vi "Destroy User Events.vi"(11 "UI Template in":refnum<class "Messages Actor.lvclass">) -> (3 "UI Template out":refnum<class "Messages Actor.lvclass">)   [LabVIEW 2020, in "Messages Actor.lvlib" / "Messages Actor.lvclass"]
uses:
  Messages Actor.lvclass
  Messages Actor.lvclass/Messages Actor.ctl
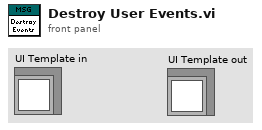
[diagram p1: front panel]
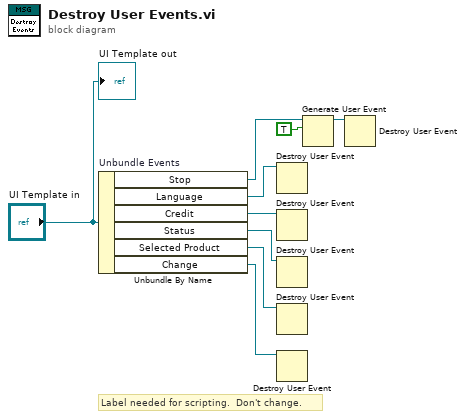
[diagram p0: block diagram]
diagram:
  # "Label needed for scripting.  Don't change."
  n1 = Unbundle By Name "Unbundle Events"("UI Template in") -> ("Stop"=w7:refnum<user-event>, "Language"=w5:refnum<user-event>, "Credit"=w4:refnum<user-event>, "Status"=w3:refnum<user-event>, "Selected Product"=w2:refnum<user-event>, "Change"=w1:refnum<user-event>)
  n2 = Destroy User Event(user event=w5) -> ()  [unwired: 1 in, 1 out]
  n3 = Destroy User Event(user event=w4) -> ()  [unwired: 1 in, 1 out]
  n4 = Destroy User Event(user event=w3) -> ()  [unwired: 1 in, 1 out]
  n5 = Destroy User Event(user event=w2) -> ()  [unwired: 1 in, 1 out]
  n6 = Destroy User Event(user event=w1) -> ()  [unwired: 1 in, 1 out]
  n7 = Generate User Event(user event=w7, event data cluster=TRUE ("event data")) -> (user event out=w8:refnum<user-event>)  [unwired: 2 in, 1 out]
  n8 = Destroy User Event(user event=w8) -> ()  [unwired: 1 in, 1 out]
  "UI Template out" <- "UI Template in"
